vi "BNT_SLContent.vi"() -> (0 "CSPP_Classes & Messages":T1(array[cluster]))   [LabVIEW 2019]
doc: "Place actor and class constants that should be included included in an application on the blockdiagramm.\n\nLizenziert unter EUPL V. 1.1"
uses:
  <vilib>/ActorFramework/Message/Message.lvclass
  BNT_SLTagMonitor/BNT_SLTagMonitor.lvclass
  C:/Users/Holger/Documents/LVP/CSPP/CSPP-Template/Packages/CSPP_Core/Actors/CSPP_BaseActor/CSPP_BaseActor.lvclass
  BNT_SLTagConnection/BNT_SLTagConnection.lvclass
  CSPP_Core/Actors/CSPP_BaseActor/CSPP_BaseActor.lvclass
  BNT_SLMsgLogger/BNT_SLMsgLogger.lvclass
panel:
  # "Place actor and class constants on the blockdiagramm."
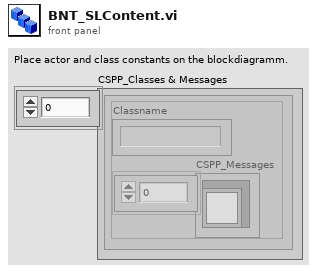
[diagram p1: front panel]
types:
  T1 = cluster{"Classname":string, "CSPP_Messages":refnum<class "Message.lvclass">[]}[]
  T2 = cluster{"class name":string, "CSPP_Messages":refnum<class "Message.lvclass">[]}
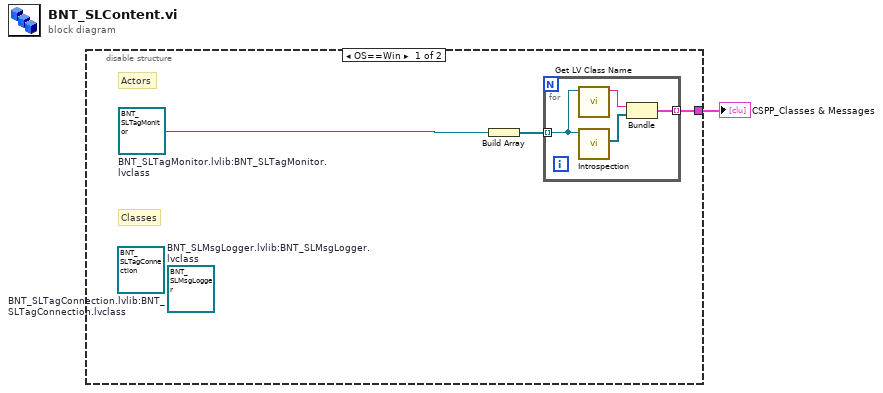
[diagram p0: block diagram]
diagram:
  n1 = disable-structure shown="OS==Win" {
    disable-tunnel: [w4 _] -> w1
    frame condition #0 (active) {
      (unwired) refnum<class "BNT_SLMsgLogger.lvclass"> refnum  # BNT_SLMsgLogger.lvlib:BNT_SLMsgLogger.lvclass
      w2 = refnum<class "BNT_SLTagMonitor.lvclass"> refnum  # BNT_SLTagMonitor.lvlib:BNT_SLTagMonitor.lvclass
      (unwired) refnum<class "BNT_SLTagConnection.lvclass"> refnum  # BNT_SLTagConnection.lvlib:BNT_SLTagConnection.lvclass
      # "Classes"
      # "Actors"
      n2 = Build Array(w2) -> (w3:refnum<class "BNT_SLTagMonitor.lvclass">[])
      n3 = for {
        tunnel: w3 -> [w8] mode=indexing
        tunnel: [w5] -> w4 mode=indexing
        n4 = call <vilib>:"Get LV Class Name.vi"("object"=w8) -> ("class name"=w7:string)  [unwired: 9 in, 1 out]
        n5 = call "Introspection.vi"("CSPP_BaseActor in"=w8) -> ("CSPP_Messages"=w6:refnum<class "Message.lvclass">[])  [unwired: 8 in, 2 out]
        n6 = Bundle("class name"=w7, "CSPP_Messages"=w6) -> (w5:T2)  [unwired: 1 in]
      }
    }
    frame condition #1 {
    }
  }
  "CSPP_Classes & Messages" <- w1
